vi "BenchC2_DEV.vi"() -> ()   [LabVIEW 2016]
uses:
  x64/Debug/BERTTA.dll
panel:
  out "element":bool
  out "Started:":string
  in  "SHUTDOWN":bool
  in  "MASTER CONTROL":bool
  in  "Tab Control":T1(tab)
  out "Output File":path caption="selected path"
  in  "Browse folder":path=path "" caption="start path"
  in  "Read Seq":bool
  in  "Save Seq":bool
  in  "Configuration file":path caption="Filename"
  in  "OK Button 2":bool
  out "Boolean":bool
  in  "User (initials)":string
  in  "Project name":string
  in  "Description":string
  out "PUMP1":bool
  out "Target amount":dbl
  out "Scale weight":dbl
  out "Amount now":dbl
  out "Flow rate":dbl
  out "Time to target":dbl format="%<%H:%M:%S>t"
  out "Current step":dbl
  out "Target":dbl
  out "Amount now":dbl
  out "Amount now":dbl
  out "Target":dbl
  out "Current step":dbl
  out "Time to target":dbl format="%<%H:%M:%S>t"
  out "Flow rate":dbl
  out "Amount now":dbl
  out "Scale weight":dbl
  out "Target amount":dbl
  out "PUMP2":bool
  out "Sensor OK 6":bool
  out "Sensor OK 5":bool
  out "Sensor OK 4":bool
  out "Sensor OK 3":bool
  in  "OK Button":bool
  in  "Add comment":string
  out "PUMP3":bool
  out "Target amount":dbl
  out "Scale weight":dbl
  out "Amount now":dbl
  out "Flow rate":dbl
  out "Time to target":dbl format="%<%H:%M:%S>t"
  out "Current step":dbl
  out "Target":dbl
  out "Amount now":dbl
  out "Tr":dbl
  out "Tj in":dbl
  out "Tj out":dbl
  out "T set":dbl
  out "Current step":i32
  out "RPM":dbl
  out "Torque 2":dbl
  out "Waveform Chart 5":dynamicdata(graph)
  out "Waveform Chart 6":dynamicdata(graph)
  out "Waveform Chart 7":dynamicdata(graph)
  in  "Tab Control 2":T2(tab)
  out "Waveform Chart 3":dynamicdata(graph)
  out "Waveform Chart 8":dynamicdata(graph)
  out "Waveform Chart 11":dynamicdata(graph)
  out "Waveform Chart 13":dynamicdata(graph)
  out "Waveform Chart 9":dynamicdata(graph)
  out "Table":string[][](table)=[["14.8.2017 18.06.59", "0,000000", "417,670000", "-0,150000", "1,000000", "22,220000", "23,366837", "23,574959", "23,985852", "23,690000", "240,000000", "4,000000", "0,000000", "397,000000", "-397,000000", "1,000000"], ["14.8.2017 18.07.06", "0,000000", "417,640000", "-0,120000", "1,000000", "22,220000", "23,763115", "23,906257", "23,985694", "23,680000", "240,000000", "4,000000", "0,000000", "397,000000", "-397,000000", "1,000000"], ["14.8.2017 18.07.13", "0,000000", "417,640000", "-0,120000", "1,000000", "22,220000", "23,965922", "24,013440", "23,984906", "23,670000", "240,000000", "4,100000", "3,000000", "397,000000", "-397,000000", "1,000000"], ["14.8.2017 18.07.21", "0,000000", "417,640000", "-0,120000", "1,000000", "22,220000", "23,943860", "23,900110", "23,987113", "23,670000", "240,000000", "4,000000", "0,000000", "397,000000", "-397,000000", "1,000000"], ["14.8.2017 18.07.28", "0,000000", "417,640000", "-0,120000", "1,000000", "22,220000", "23,736328", "23,600018", "23,989004", "23,660000", "240,000000", "4,000000", "0,000000", "397,000000", "-397,000000", "1,000000"], ["14.8.2017 18.07.36", "0,000000", "417,640000", "-0,120000", "1,000000", "22,220000", "23,480910", "23,324538", "23,991053", "23,660000", "240,000000", "4,000000", "0,000000", "397,000000", "-397,000000", "1,000000"], ["14.8.2017 18.07.43", "0,000000", "417,640000", "-0,120000", "2,000000", "22,220000", "23,195579", "23,008270", "23,999093", "23,650000", "240,000000", "4,000000", "0,000000", "397,000000", "-397,000000", "1,000000"], ["14.8.2017 18.07.51", "0,000000", "417,650000", "-417,650000", "1,000000", "22,220000", "22,862541", "22,649021", "24,003979", "23,650000", "240,000000", "4,000000", "0,000000", "397,000000", "-397,000000", "2,000000"], ["14.8.2017 18.07.58", "0,000000", "417,640000", "0,010000", "1,000000", "22,220000", "22,541353", "22,354878", "24,005398", "23,650000", "240,000000", "4,000000", "0,000000", "397,000000", "-397,000000", "1,000000"], ["14.8.2017 18.08.06", "0,000000", "417,640000", "0,010000", "1,000000", "22,220000", "22,347931", "22,253738", "24,007605", "23,640000", "240,000000", "4,100000", "0,000000", "397,000000", "-397,000000", "1,000000"], ["14.8.2017 18.08.13", "0,000000", "417,640000", "0,010000", "1,000000", "22,220000", "22,329030", "22,302102", "24,006028", "23,640000", "240,000000", "4,000000", "0,000000", "395,820000", "-395,820000", "1,000000"], ["14.8.2017 18.08.20", "0,000000", "417,640000", "0,010000", "1,000000", "22,220000", "22,466849", "22,511320", "24,002403", "23,630000", "240,000000", "4,000000", "0,000000", "395,830000", "-0,010000", "1,000000"], ["14.8.2017 18.08.28", "0,000000", "417,640000", "0,010000", "1,000000", "22,220000", "22,707062", "22,835101", "24,000984", "23,620000", "240,000000", "4,000000", "0,000000", "395,830000", "-0,010000", "1,000000"], ["14.8.2017 18.08.35", "0,000000", "417,640000", "0,010000", "1,000000", "22,220000", "23,054104", "23,232979", "24,001299", "23,600000", "240,000000", "4,000000", "0,000000", "395,830000", "-0,010000", "1,000000"], ["14.8.2017 18.08.43", "0,000000", "417,640000", "0,010000", "1,000000", "22,220000", "23,412371", "23,522793", "24,002560", "23,590000", "240,000000", "4,000000", "0,000000", "395,820000", "0,000000", "1,000000"], ["14.8.2017 18.08.51", "0,000000", "417,640000", "0,010000", "1,000000", "22,220000", "23,596247", "23,656125", "24,003821", "23,580000", "240,000000", "4,000000", "0,000000", "395,820000", "0,000000", "1,000000"]]
  in  "X scale":i64(slide)=50 scale=0.0..100.0
  in  "Tr/Tj mode selector 2":bool=TRUE
  in  "Tr/Tj mode selector":bool=TRUE
  out "Boolean 4":bool
  out "Boolean 3":bool
  out "Boolean 2":bool
  in  "Reset 6":bool
  in  "Manual/Ramp":bool=TRUE
  in  "Array":dbl[][](array[numeric])=[[20.0, 0.0], [20.0, 0.0], [20.0, 0.0]]
  in  "?":bool
  in  "Time":dbl format="Time to target (min):                %#_g"
  out "Current temp":dbl format="Current temperature (S1):   %#_6g"
  in  "OK Button 3":bool
  out "Sensor OK":bool
  in  "T fail":dbl=20.0 format="Failsafe temperature:              %#_g"
  in  "Setpoint":dbl=20.0 format="Temperature target:                %#_6g"
  out "Waveform Chart":dynamicdata(graph)
  out "T external 2":dbl format="Current temp S2:    %#_g"
  in  "UPDATE TEMP":bool
  out "Waveform Chart 2":dbl(graph)
  in  "Tube select":u32(ring) items=["Purple tube", "Yellow tube", " White tube"]
  out "Led11 5":bool
  out "RPM":dbl format="%_4f"
  out "Led5 3":bool
  out "Led4 3":bool
  out "Led3 3":bool
  out "Led2 3":bool
  out "Led1 3":bool
  in  "PumpSeq 4":dbl[][](array[numeric])=[[0.0, 0.0, 0.0, 0.0, 0.0, 0.0, 0.0, 0.0, 0.0, 0.0], [0.0, 0.0, 0.0, 0.0, 0.0, 0.0, 0.0, 0.0, 0.0, 0.0], [0.0, 0.0, 0.0, 0.0, 0.0, 0.0, 0.0, 0.0, 0.0, 0.0], [0.0, 0.0, 0.0, 0.0, 0.0, 0.0, 0.0, 0.0, 0.0, 0.0], [0.0, 0.0, 0.0, 0.0, 0.0, 0.0, 0.0, 0.0, 0.0, 0.0], [0.0, 0.0, 0.0, 0.0, 0.0, 0.0, 0.0, 0.0, 0.0, 0.0], [0.0, 0.0, 0.0, 0.0, 0.0, 0.0, 0.0, 0.0, 0.0, 0.0], [0.0, 0.0, 0.0, 0.0, 0.0, 0.0, 0.0, 0.0, 0.0, 0.0], [0.0, 0.0, 0.0, 0.0, 0.0, 0.0, 0.0, 0.0, 0.0, 0.0], [0.0, 0.0, 0.0, 0.0, 0.0, 0.0, 0.0, 0.0, 0.0, 0.0]]
  in  "?":bool
  out "Flow rate (g/min)":dbl
  out "Scale reading":dbl
  out "Step amount now":dbl
  in  "Grams / min":dbl
  out "Waveform Chart 14":dynamicdata(graph)
  in  "?":bool
  out "Total amount now":dbl
  out "Led11 4":bool
  in  "Reset 5":bool
  out "Elapsed / step":dbl format="%<%H:%M:%S>t"
  out "Time to target":dbl format="%<%H:%M:%S>t"
  in  "OK Button 4":bool
  out "Led11":bool
  out "RPM":dbl format="%_4f"
  out "Led10":bool
  out "Led9":bool
  out "Led8":bool
  out "Led7":bool
  out "Led6":bool
  out "Led5":bool
  out "Led4":bool
  out "Led3":bool
  out "Led2":bool
  out "Led1":bool
  in  "PumpSeq 2":dbl[][](array[numeric])=[[0.0, 0.0, 0.0, 0.0, 0.0, 0.0, 0.0, 0.0, 0.0, 0.0], [0.0, 0.0, 0.0, 0.0, 0.0, 0.0, 0.0, 0.0, 0.0, 0.0], [0.0, 0.0, 0.0, 0.0, 0.0, 0.0, 0.0, 0.0, 0.0, 0.0], [0.0, 0.0, 0.0, 0.0, 0.0, 0.0, 0.0, 0.0, 0.0, 0.0], [0.0, 0.0, 0.0, 0.0, 0.0, 0.0, 0.0, 0.0, 0.0, 0.0], [0.0, 0.0, 0.0, 0.0, 0.0, 0.0, 0.0, 0.0, 0.0, 0.0], [0.0, 0.0, 0.0, 0.0, 0.0, 0.0, 0.0, 0.0, 0.0, 0.0], [0.0, 0.0, 0.0, 0.0, 0.0, 0.0, 0.0, 0.0, 0.0, 0.0], [0.0, 0.0, 0.0, 0.0, 0.0, 0.0, 0.0, 0.0, 0.0, 0.0], [0.0, 0.0, 0.0, 0.0, 0.0, 0.0, 0.0, 0.0, 0.0, 0.0]]
  in  "?":bool
  out "Flow rate (g/min)":dbl
  out "Scale reading":dbl
  out "Step amount now":dbl
  in  "Grams / min":dbl
  out "Waveform Chart 10":dynamicdata(graph)
  in  "?":bool
  out "Total amount now":dbl
  out "Led11":bool
  in  "Reset 3":bool
  out "Elapsed / step":i32
  out "Time to target":dbl format="%<%H:%M:%S>t"
  in  "OK Button 5":bool
  out "Led11 3":bool
  out "RPM":dbl format="%_4f"
  out "Led10 2":bool
  out "Led9 2":bool
  out "Led8 2":bool
  out "Led7 2":bool
  out "Led6 2":bool
  out "Led5 2":bool
  out "Led4 2":bool
  out "Led3 2":bool
  out "Led2 2":bool
  out "Led1 2":bool
  in  "PumpSeq 3":dbl[][](array[numeric])=[[0.0, 0.0, 0.0, 0.0, 0.0, 0.0, 0.0, 0.0, 0.0, 0.0], [0.0, 0.0, 0.0, 0.0, 0.0, 0.0, 0.0, 0.0, 0.0, 0.0], [0.0, 0.0, 0.0, 0.0, 0.0, 0.0, 0.0, 0.0, 0.0, 0.0], [0.0, 0.0, 0.0, 0.0, 0.0, 0.0, 0.0, 0.0, 0.0, 0.0], [0.0, 0.0, 0.0, 0.0, 0.0, 0.0, 0.0, 0.0, 0.0, 0.0], [0.0, 0.0, 0.0, 0.0, 0.0, 0.0, 0.0, 0.0, 0.0, 0.0], [0.0, 0.0, 0.0, 0.0, 0.0, 0.0, 0.0, 0.0, 0.0, 0.0], [0.0, 0.0, 0.0, 0.0, 0.0, 0.0, 0.0, 0.0, 0.0, 0.0], [0.0, 0.0, 0.0, 0.0, 0.0, 0.0, 0.0, 0.0, 0.0, 0.0], [0.0, 0.0, 0.0, 0.0, 0.0, 0.0, 0.0, 0.0, 0.0, 0.0]]
  in  "?":bool
  out "Flow rate (g/min)":dbl
  out "Scale reading":dbl
  out "Step amount now":dbl
  in  "Grams / min":dbl
  out "Waveform Chart 12":dynamicdata(graph)
  in  "?":bool
  out "Total amount now":dbl
  out "Led11 2":bool
  in  "Reset 4":bool
  out "Elapsed / step":i32
  out "Time to target":dbl format="%<%H:%M:%S>t"
  in  "OK Button 6":bool
  in  "?":bool
  in  "Scale port":dbl=5.0
  out "Waveform Chart 15":dynamicdata(graph)
  in  "?":bool
  in  "OK Button 8":bool
  in  "Remote / Manual":bool
  in  "Set RPM":i32
  out "RPM":dbl
  out "Torque":dbl
  out "Waveform Chart 4":dynamicdata(graph)
  in  "OK Button 7":bool
  out "PortDev out":dbl[](array[numeric])
  in  "Save PortDev":bool
  out "PortDev in":dbl[](array[numeric])
  in  "dev1":i32
  in  "dev2":i32
  in  "dev3":i32
  in  "dev4":i32
  in  "dev5":i32
  in  "dev6":i32
  in  "dev8":i32
  in  "port1":i32
  in  "port2":i32
  in  "port3":i32
  in  "port4":i32
  in  "port5":i32
  in  "port6":i32
  in  "port7":i32
  in  "port8":i32
  in  "dev7":i32
  in  "Treshold (T/C)":dbl=0.5
  out "DAQ 9217 (PT100)":errorcluster
  out "Config File":dbl[][](array[numeric])
  in  "Temp Control":tag="cDAQ9188XT-1C3BF2FMod1"
  in  "PAM Control":tag="cDAQ9188XT-1C3BF2FMod7"
  # "Temperature sensor:"
  # "Manual control:"
  # "PUMP & SCALE 1"
  # "STEP"
  # "TOTAL"
  # "PUMP & SCALE 2"
  # "STEP"
  # "TOTAL"
  # "PUMP & SCALE 3"
  # "STEP"
  # "TOTAL"
  # "Temperature control parameter"
  # "Secondary temperature sensor"
  # "Temp target"
  # "Time target"
  # "Grams    /   min"
  # "End of sequence"
  # "Manual control"
  # "Grams    /   min"
  # "End of sequence"
  # "Manual control"
  # "Grams    /   min"
  # "End of sequence"
  # "Manual control"
  # "PAM control"
  # "dev1 and dev2 always to port1 and 2\nport1 = port2 = Lauda\n\ndev3 and dev4 always to port3 and port4\nport3 = port4 = Heidolph"
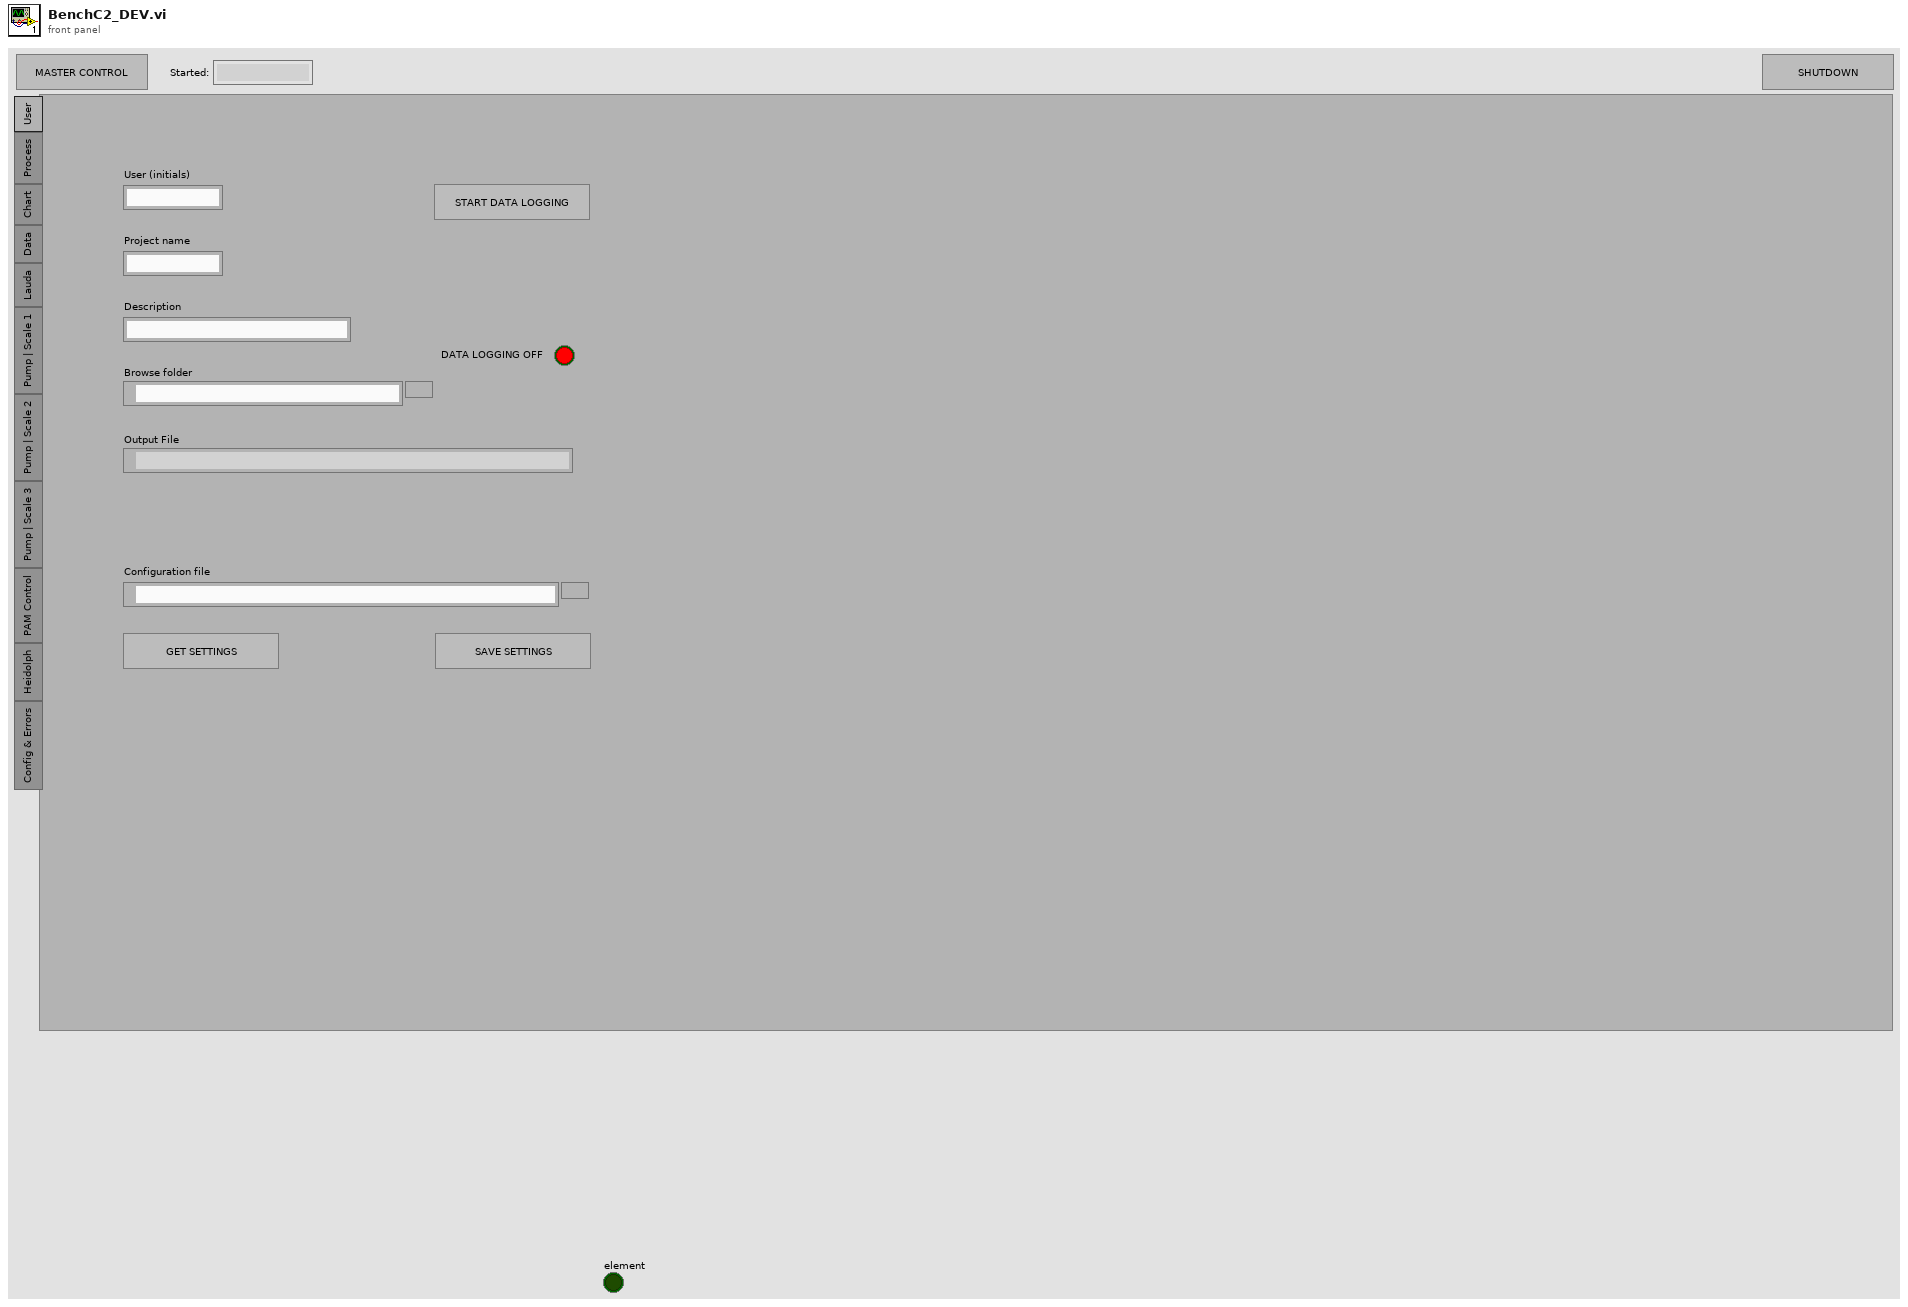
[diagram p1: front panel]
types:
  T1 = enum32{"User", "Process", "Chart", "Data", "Lauda", "Pump | Scale 1", "Pump | Scale 2", "Pump | Scale 3", "PAM Control", "Heidolph", "Config & Errors"}
  T2 = enum32{"Temperatures", "Scale / Pump 1", "Scale / Pump 2", "Scale / Pump 3", "RPM / torque"}
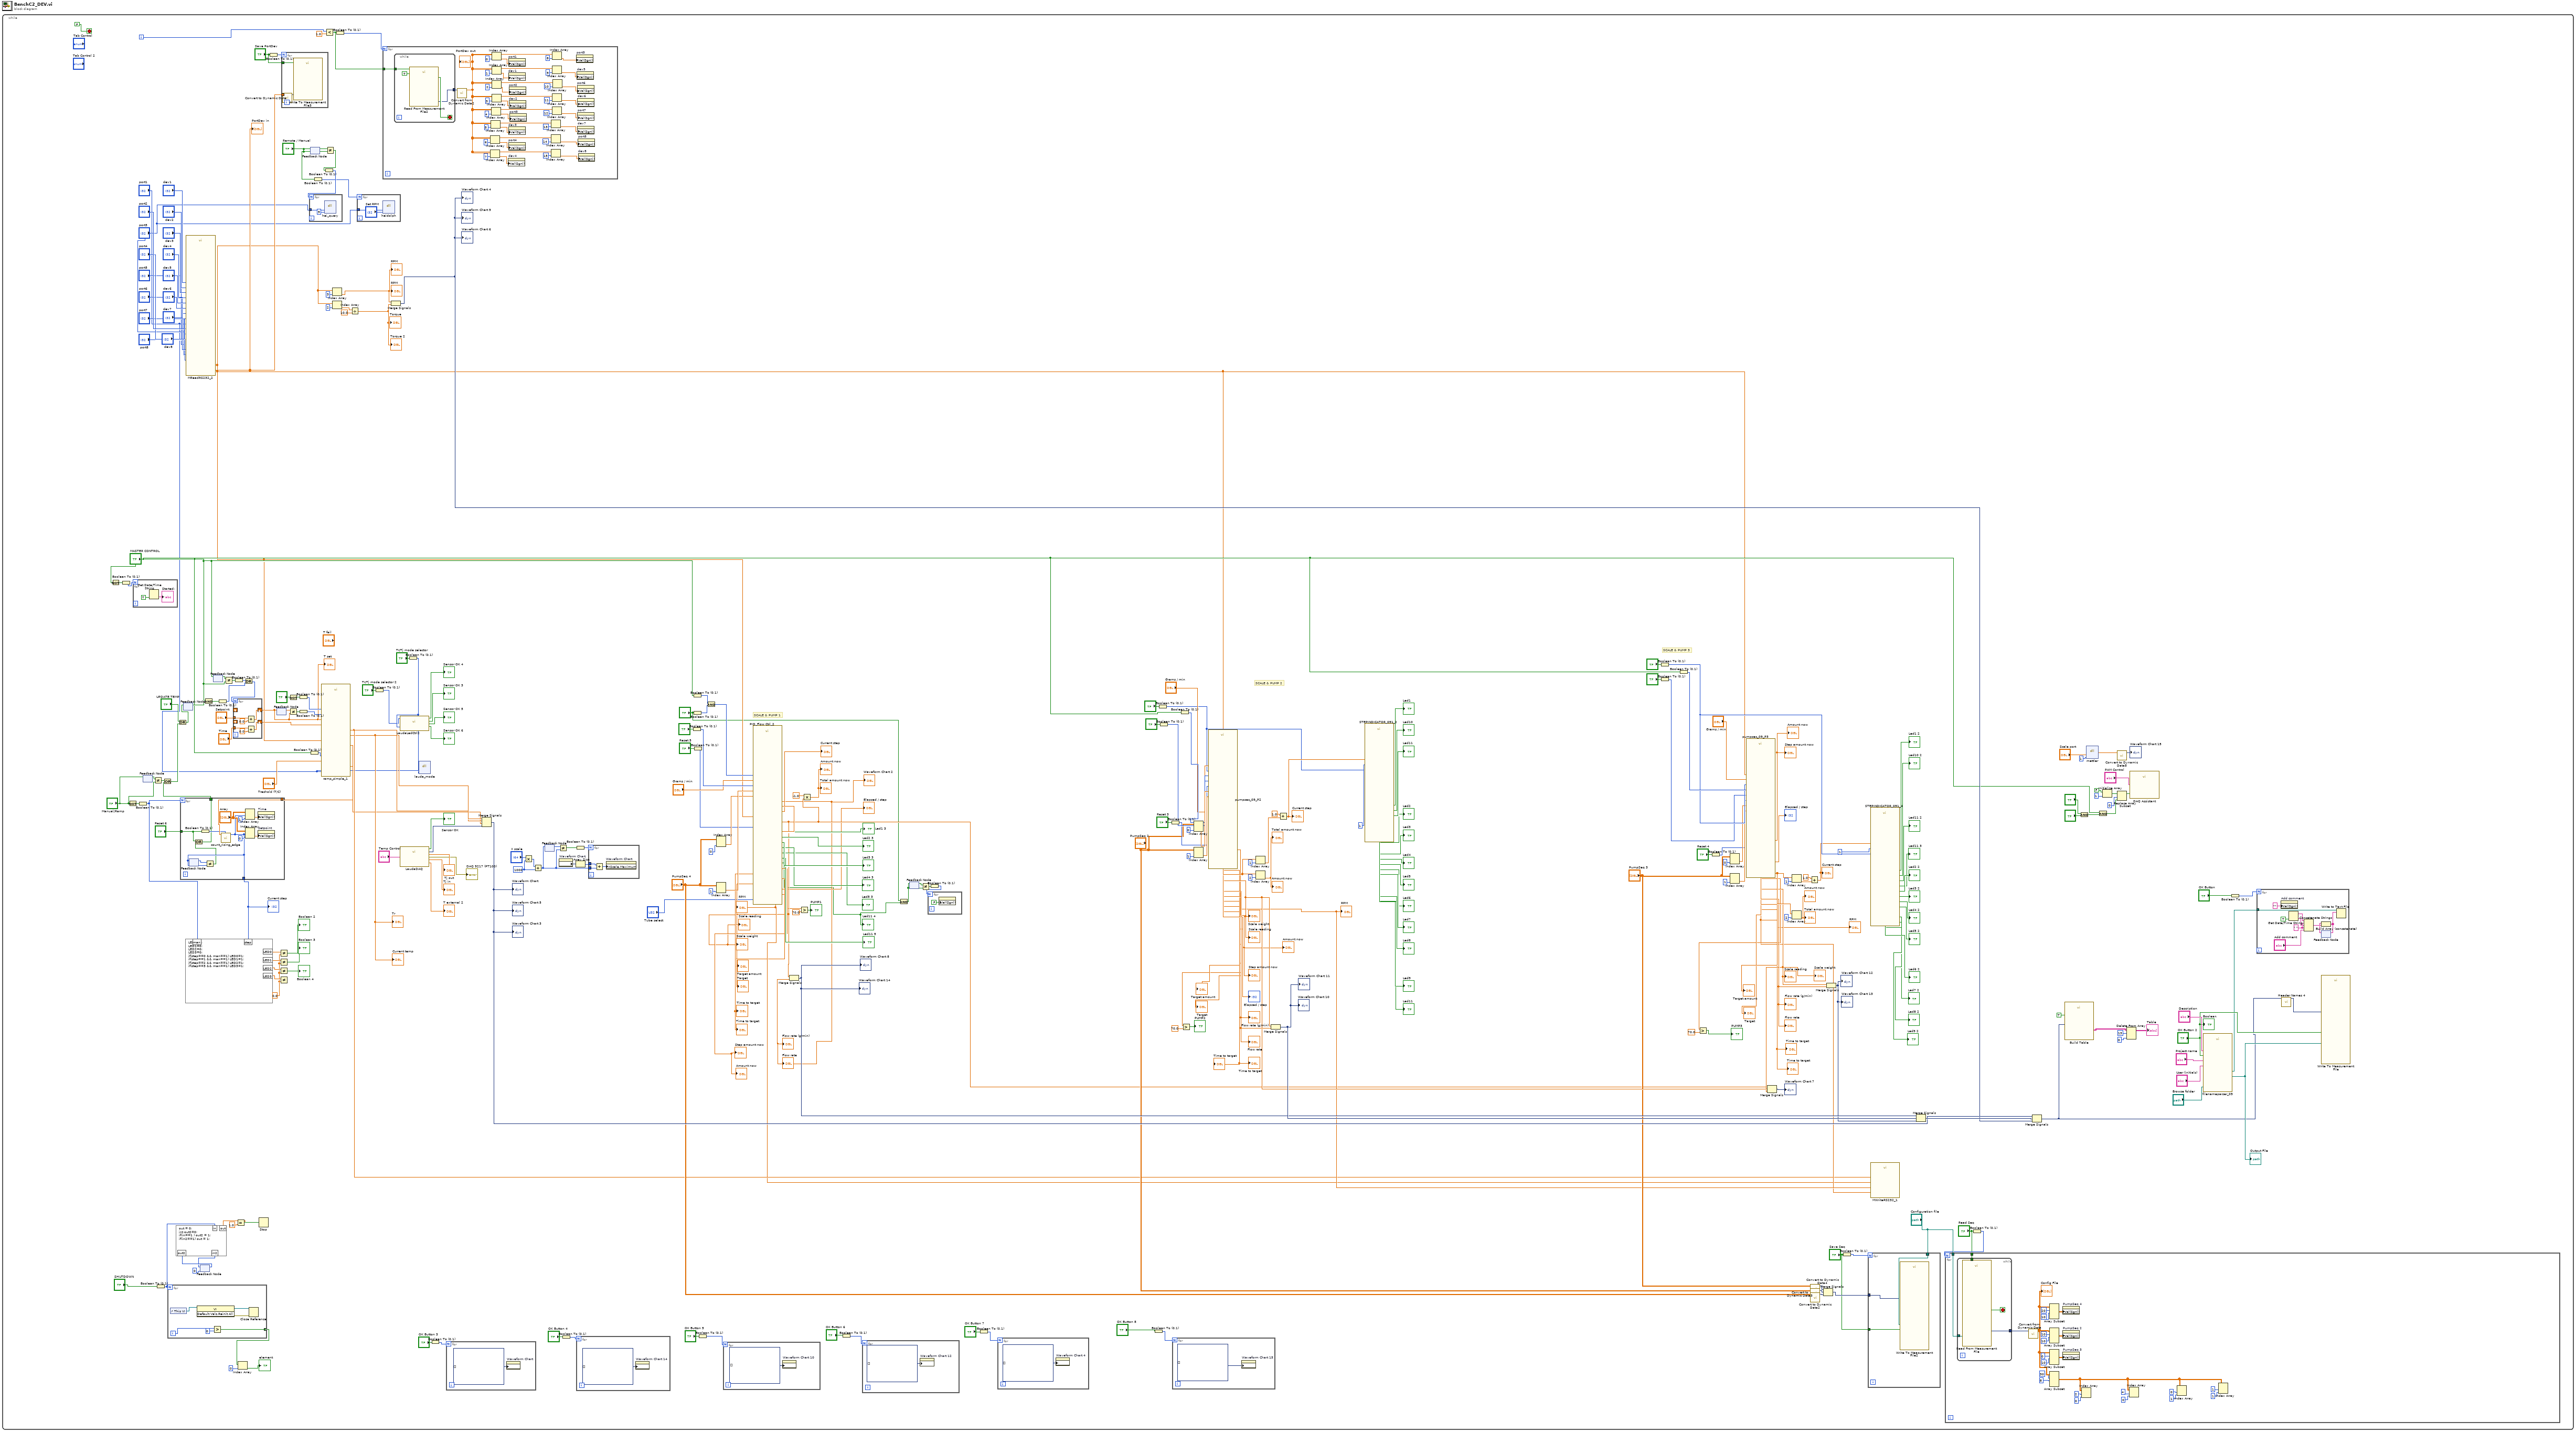
[diagram p0: block diagram]
diagram:
  n1 = while {
    i -> [w110]
    stop <- FALSE stop-if-true
    w42 = i64 1000 ("y")
    w96 = 0.0 ("y")
    # "SCALE & PUMP 1"
    # "SCALE & PUMP 3"
    # "SCALE & PUMP 2"
    n2 = Not(x="MASTER CONTROL") -> (.not. x?=w297:bool)
    n3 = Boolean To (0,1)(Boolean=w297) -> (0, 1=w298:i16)
    n4 = Not(x="Manual/Ramp") -> (.not. x?=w103:bool)
    n5 = for {
      N: w298 -> [_]
      n6 = Get Date/Time String(want seconds? (F)=TRUE) -> (time string=→"Started:":string)  [unwired: 2 in, 1 out]
    }
    n7 = Boolean To (0,1)(Boolean=w103) -> (0, 1=w86:i16)
    n8 = feedback #1() -> (w92:bool)  [unwired: 1 in]
    n9 = feedback-in #1("Manual/Ramp") -> ()
    n10 = Not Equal?(x=w92, y="Manual/Ramp") -> (x != y?=w89:bool)
    n11 = Boolean To (0,1)(Boolean="SHUTDOWN") -> (0, 1=w282:i16)
    n12 = for {
      N: w282 -> [_]
      tunnel: [w418] -> w296 mode=indexing
      i -> [w420]
      n13 = control-ref of="This VI"() -> (w423:refnum<vi>)
      n14 = invoke class="VI" method="Default Vals.Reinit All"(reference=w423) -> (reference out=w421:refnum<vi>, error out=w422:errorcluster)  [unwired: 2 in, 1 out]
      n15 = Greater?(x=w420, y=0) -> (0:w418:bool)
      n16 = Close Reference(reference=w421, error in (no error)=w422) -> ()  [unwired: 1 out]
    }
    n17 = feedback #2() -> (w84:bool)  [unwired: 1 in]
    n18 = call "MReadRS232_2.vi"("port1"="port1", "dev1"="dev1", "port2"="port2", "dev2"="dev2", "port3"="port3", "dev7"="dev7", "dev8"="dev8", "port7"="port7", "port8"="port8", "dev5"="dev5", "port5"="port5", "dev4"="dev4", "dev6"="dev6", "port6"="port6", "port4"="port4", "dev3"="dev3") -> ("output array"=w114:dbl[], "params"=w30:dbl[])  [unwired: 2 in]
    "PortDev in" <- w114
    n19 = feedback #3(0) -> (w280:i32)
    n20 = formula code="out = 0;\nint out2=0;\nif(in==1 ) out2 = 1;\nif(in2==1) out = 1;"("in"=w282, "in2"=w280) -> ("out"=w284:dbl, "out2"=w281:i32)
    n21 = feedback-in #3(w281) -> ()
    n22 = And(x="MASTER CONTROL", y=w84) -> (x .and. y?=w140:bool)
    n23 = feedback #4() -> (w132:bool)  [unwired: 1 in]
    n24 = feedback-in #4("MASTER CONTROL") -> ()
    n25 = Boolean To (0,1)(Boolean=w140) -> (0, 1=w130:i16)
    n26 = Not Equal?(x=w132, y="MASTER CONTROL") -> (x != y?=w131:bool)
    n27 = Boolean To (0,1)(Boolean=w131) -> (0, 1=w129:i16)
    n28 = Equal?(x=w284, y=1.0) -> (x = y?=w283:bool)
    n29 = Index Array(array=w296, index=0) -> (element=→"element":bool)
    n30 = Or(x=w129, y=w130) -> (x .or. y?=w128:i16)
    n31 = for {
      N: w128 -> [_]
      tunnel: "Time" -> [w370]
      shift-right: [w369] -> w141
      shift-left: _ -> [_]
      tunnel: "Setpoint" -> [w367]
      shift-right: [w366] -> w51
      shift-left: _ -> [_]
      n32 = Add(x=w367, y=0.0) -> (x+y=w366:dbl)
      n33 = Add(x=w370, y=0.0) -> (x+y=w369:dbl)
    }
    "T set" <- w51
    n34 = Stop(stop? (T)=w283) -> ()
    n35 = Boolean To (0,1)(Boolean="Save PortDev") -> (0, 1=w113:i16)
    n36 = feedback-in #5(w51) -> ()
    n37 = feedback #5() -> (w139:dbl)  [unwired: 1 in]
    n38 = for {
      N: w113 -> [_]
      tunnel: w114 -> [w365]
      tunnel: "Save PortDev" -> [w363]
      n39 = call "Convert to Dynamic Data"("Array"=w365) -> ("Dynamic Data Type"=w364:dynamicdata)  [unwired: 3 in]
      n40 = call "Write To Measurement File3"("Signals"=w364, "Reset"=w363) -> ()  [unwired: 15 in, 3 out]
    }
    n41 = Not(x="?") -> (.not. x?=w135:bool)
    n42 = Not Equal?(x=w139, y=w51) -> (x != y?=w138:bool)
    n43 = Boolean To (0,1)(Boolean=w135) -> (0, 1=w137:i16)
    n44 = Boolean To (0,1)(Boolean=w138) -> (0, 1=w133:i16)
    n45 = Boolean To (0,1)(Boolean="MASTER CONTROL") -> (0, 1=w134:i16)
    n46 = feedback-in #6("Remote / Manual") -> ()
    n47 = feedback #6() -> (w81:bool)  [unwired: 1 in]
    n48 = Boolean To (0,1)(Boolean="Remote / Manual") -> (0, 1=w79:i16)
    n49 = call "ramp_simple_1.vi"("pause"=w137, "time_set"=w141, "array"=w30, "reset"=w133, "master"=w134, "T_sp"=w51, "treshold"="Treshold (T/C)", "port"="port1") -> ("Tin"=w144:dbl, "Tr"=w145:dbl, "target_reached"=w101:dbl, "T control"=w146:dbl)  [unwired: 3 in, 1 out]
    "Tr" <- w145
    "Current temp" <- w145
    n50 = for {
      N: w86 -> [_]
      tunnel: w101 -> [w322]
      tunnel: [w312] -> w90
      tunnel: "Reset 6" -> [w314]
      tunnel: [w315] -> w52
      n51 = feedback #7() -> (w316:i32)  [unwired: 1 in]
      n52 = Boolean To (0,1)(Boolean=w314) -> (0, 1=w317:i16)
      n53 = call "count_rising_edge.vi"("reset"=w317, "target_reached"=w322) -> ("element 2"=w315:i32)  [unwired: 9 in]
      n54 = feedback-in #7(w315) -> ()
      n55 = Not Equal?(x=w316, y=w315) -> (x != y?=w313:bool)
      n56 = Or(x=w314, y=w313) -> (x .or. y?=w312:bool)
      n57 = Index Array(array="Array", index (row)=w315, index (col)=1 ("disabled index (col)")) -> (element=w318:dbl)
      n58 = Index Array(array="Array", index (row)=w315, index (col)=0 ("disabled index (col)")) -> (element=w319:dbl)
      n59 = property on="Time" class="DigNum (strict)"("Val(Sgnl)"=w318) -> ()  [unwired: 2 in, 2 out]
      n60 = property on="Setpoint" class="DigNum (strict)"("Val(Sgnl)"=w319) -> ()  [unwired: 2 in, 2 out]
    }
    "Current step" <- w52
    n61 = Or(x=w89, y=w90) -> (x .or. y?=w88:bool)
    n62 = Or(x="UPDATE TEMP", y=w88) -> (x .or. y?=w85:bool)
    n63 = feedback-in #2(w85) -> ()
    n64 = formula code="LED0=0;\nLED1=0;\nLED2=0;\nLED3=0;\nif(step==0 && man==1) LED0=1;\nif(step==1 && man==1) LED1=1;\nif(step==2 && man==1) LED2=1;\nif(step==3 && man==1) LED3=1;"("step"=w52, "man"=w86) -> ("LED0"=w100:dbl, "LED1"=w99:dbl, "LED2"=w98:dbl, "LED3"=w97:dbl)
    n65 = Not Equal?(x=w100, y=w96) -> (x != y?=→"Boolean 2":bool)
    n66 = Not Equal?(x=w99, y=w96) -> (x != y?=→"Boolean 3":bool)
    n67 = Not Equal?(x=w98, y=w96) -> (x != y?=→"Boolean 4":bool)
    n68 = Not Equal?(x=w97, y=w96) -> ()  [unwired: 1 out]
    n69 = Less?(x=w110, y=1.0) -> (x < y?=w108:bool)
    n70 = Not Equal?(x=w81, y="Remote / Manual") -> (x != y?=w80:bool)
    n71 = Boolean To (0,1)(Boolean=w80) -> (0, 1=w82:i16)
    n72 = for {
      N: w82 -> [_]
      tunnel: "port3" -> [w310]
      n73 = dll-call lib="C:/Users/shresplab/OneDrive - Kemira Oyj/Documents/GitHub/Bertta/BERTTA/x64/Debug/BERTTA.dll" fn="hei_query"("port"=w310, "q"=5) -> ()  [unwired: 6 in, 2 out]
    }
    n74 = Index Array(array=w30, index=3) -> (element=w74:dbl)
    "RPM" <- w74
    "RPM" <- w74
    n75 = Index Array(array=w30, index=2) -> (element=w76:dbl)
    n76 = Boolean To (0,1)(Boolean=w108) -> (0, 1=w109:i16)
    n77 = Divide(x=w76, y=10.0) -> (x/y=w73:dbl)
    "Torque" <- w73
    "Torque 2" <- w73
    n78 = for {
      N: w79 -> [_]
      tunnel: "port3" -> [w308]
      n79 = dll-call lib="C:/Users/shresplab/OneDrive - Kemira Oyj/Documents/GitHub/Bertta/BERTTA/x64/Debug/BERTTA.dll" fn="heidolph"("port"=w308, "speed"="Set RPM") -> ()  [unwired: 6 in, 2 out]
    }
    n80 = Boolean To (0,1)(Boolean="Tr/Tj mode selector 2") -> (0, 1=w46:i16)
    n81 = for {
      N: w109 -> [_]
      tunnel: w108 -> [w358]
      n82 = while {
        tunnel: [w361] -> w357
        tunnel: w358 -> [w359]
        stop <- w362 stop-if-true
        n83 = call "Read From Measurement File2"("Enable"=TRUE, "Reset"=w359) -> ("Signals"=w361:dynamicdata, "EOF?"=w362:bool)  [unwired: 4 in, 4 out]
      }
      n84 = call "Convert from Dynamic Data2"("Dynamic Data Type"=w357) -> ("Array"=w340:dbl[])  [unwired: 3 in]
      "PortDev out" <- w340
      n85 = Index Array(array=w340, index=6) -> (element=w333:dbl)
      n86 = Index Array(array=w340, index=7) -> (element=w332:dbl)
      n87 = Index Array(array=w340, index=5) -> (element=w334:dbl)
      n88 = Index Array(array=w340, index=4) -> (element=w335:dbl)
      n89 = Index Array(array=w340, index=0) -> (element=w339:dbl)
      n90 = Index Array(array=w340, index=1) -> (element=w338:dbl)
      n91 = Index Array(array=w340, index=3) -> (element=w336:dbl)
      n92 = Index Array(array=w340, index=2) -> (element=w337:dbl)
      n93 = property on="dev4" class="DigNum (strict)"("Val(Sgnl)"=w332) -> ()  [unwired: 2 in, 2 out]
      n94 = property on="dev3" class="DigNum (strict)"("Val(Sgnl)"=w334) -> ()  [unwired: 2 in, 2 out]
      n95 = property on="port4" class="DigNum (strict)"("Val(Sgnl)"=w333) -> ()  [unwired: 2 in, 2 out]
      n96 = property on="port1" class="DigNum (strict)"("Val(Sgnl)"=w339) -> ()  [unwired: 2 in, 2 out]
      n97 = property on="dev1" class="DigNum (strict)"("Val(Sgnl)"=w338) -> ()  [unwired: 2 in, 2 out]
      n98 = property on="port2" class="DigNum (strict)"("Val(Sgnl)"=w337) -> ()  [unwired: 2 in, 2 out]
      n99 = property on="dev2" class="DigNum (strict)"("Val(Sgnl)"=w336) -> ()  [unwired: 2 in, 2 out]
      n100 = property on="port3" class="DigNum (strict)"("Val(Sgnl)"=w335) -> ()  [unwired: 2 in, 2 out]
      n101 = Index Array(array=w340, index=14) -> (element=w325:dbl)
      n102 = Index Array(array=w340, index=15) -> (element=w324:dbl)
      n103 = Index Array(array=w340, index=13) -> (element=w326:dbl)
      n104 = Index Array(array=w340, index=12) -> (element=w327:dbl)
      n105 = Index Array(array=w340, index=8) -> (element=w331:dbl)
      n106 = Index Array(array=w340, index=9) -> (element=w330:dbl)
      n107 = Index Array(array=w340, index=11) -> (element=w328:dbl)
      n108 = Index Array(array=w340, index=10) -> (element=w329:dbl)
      n109 = property on="port5" class="DigNum (strict)"("Val(Sgnl)"=w331) -> ()  [unwired: 2 in, 2 out]
      n110 = property on="dev5" class="DigNum (strict)"("Val(Sgnl)"=w330) -> ()  [unwired: 2 in, 2 out]
      n111 = property on="port6" class="DigNum (strict)"("Val(Sgnl)"=w329) -> ()  [unwired: 2 in, 2 out]
      n112 = property on="dev6" class="DigNum (strict)"("Val(Sgnl)"=w328) -> ()  [unwired: 2 in, 2 out]
      n113 = property on="port7" class="DigNum (strict)"("Val(Sgnl)"=w327) -> ()  [unwired: 2 in, 2 out]
      n114 = property on="dev7" class="DigNum (strict)"("Val(Sgnl)"=w326) -> ()  [unwired: 2 in, 2 out]
      n115 = property on="port8" class="DigNum (strict)"("Val(Sgnl)"=w325) -> ()  [unwired: 2 in, 2 out]
      n116 = property on="dev8" class="DigNum (strict)"("Val(Sgnl)"=w324) -> ()  [unwired: 2 in, 2 out]
    }
    n117 = Merge Signals(w74, w73) -> (w72:dynamicdata)
    "Waveform Chart 4" <- w72
    "Waveform Chart 6" <- w72
    "Waveform Chart 9" <- w72
    n118 = call "LaudaDAQ.vi"("device name"="Temp Control") -> ("error out"=→"DAQ 9217 (PT100)":errorcluster, 1:"Tj out"=→"Tj out":dbl, "data"=w202:dynamicdata, "Sensor OK"=→"Sensor OK":bool, 4:"Tj out"=→"Tj in":dbl, "T external 2"=→"T external 2":dbl)  [unwired: 5 in]
    n119 = Boolean To (0,1)(Boolean="Tr/Tj mode selector") -> (0, 1=w48:i16)
    n120 = call "LaudaLedCtrl2.vi"("ctrl_mode"=w48, "T ext / T ext in"=w46) -> ("Sensor OK 5"=→"Sensor OK 5":bool, "Sensor OK 3"=→"Sensor OK 3":bool, "Sensor OK 4"=→"Sensor OK 4":bool, "Sensor OK 6"=→"Sensor OK 6":bool)  [unwired: 6 in]
    n121 = dll-call lib="C:/Users/shresplab/OneDrive - Kemira Oyj/Documents/GitHub/Bertta/BERTTA/x64/Debug/BERTTA.dll" fn="lauda_mode"("port"="port1", "mode"=w48) -> ()  [unwired: 6 in, 2 out]
    n122 = Boolean To (0,1)(Boolean="OK Button 3") -> (0, 1=w157:i16)
    n123 = for {
      N: w157 -> [_]
      n124 = property on="Waveform Chart" class="WFChart (strict)"("History Data"=dynamicdata[] []) -> ()  [unwired: 2 in, 2 out]
    }
    n125 = Merge Signals(w146, w145, w144, w202) -> (w203:dynamicdata)
    "Waveform Chart 3" <- w203
    "Waveform Chart" <- w203
    "Waveform Chart 5" <- w203
    n126 = Multiply(x="X scale", y=w42) -> (x*y=w43:i64)
    n127 = Add(x=w43, y=w42) -> (x+y=w38:i64)
    n128 = feedback-in #8(w38) -> ()
    n129 = feedback #8() -> (w41:i64)  [unwired: 1 in]
    n130 = Not Equal?(x=w41, y=w38) -> (x != y?=w40:bool)
    n131 = property on="Waveform Chart" class="WFChart (strict)"() -> ("History Data"=w45:dynamicdata[])  [unwired: 2 in, 2 out]
    n132 = Boolean To (0,1)(Boolean="OK Button 4") -> (0, 1=w155:i16)
    n133 = Boolean To (0,1)(Boolean=w40) -> (0, 1=w37:i16)
    n134 = Array Size(array=w45) -> (size(s)=w39:i32)
    n135 = for {
      N: w155 -> [_]
      n136 = property on="Waveform Chart 14" class="WFChart (strict)"("History Data"=dynamicdata[] []) -> ()  [unwired: 2 in, 2 out]
    }
    n137 = for {
      N: w37 -> [_]
      tunnel: w39 -> [w306]
      tunnel: w38 -> [w305]
      n138 = Add(x=w306, y=w305) -> (x+y=w304:i64)
      n139 = property on="Waveform Chart" class="WFChart (strict)"("XScale.Maximum"=w304) -> ()  [unwired: 2 in, 2 out]
    }
    n140 = Boolean To (0,1)(Boolean="?") -> (0, 1=w36:i16)
    n141 = Boolean To (0,1)(Boolean="?") -> (0, 1=w7:i16)
    n142 = Boolean To (0,1)(Boolean="MASTER CONTROL") -> (0, 1=w34:i16)
    n143 = Boolean To (0,1)(Boolean="Reset 5") -> (0, 1=w28:i16)
    n144 = Boolean To (0,1)(Boolean="OK Button 5") -> (0, 1=w153:i16)
    n145 = And(x=w34, y=w7) -> (x .and. y?=w33:i16)
    n146 = Index Array(array="PumpSeq 4", index (col)=0) -> (element=w31:dbl[])  [unwired: 1 in]
    n147 = Index Array(array="PumpSeq 4", index (col)=1) -> (element=w32:dbl[])  [unwired: 1 in]
    n148 = for {
      N: w153 -> [_]
      n149 = property on="Waveform Chart 10" class="WFChart (strict)"("History Data"=dynamicdata[] []) -> ()  [unwired: 2 in, 2 out]
    }
    n150 = call "PID_Flow Ctrl_2.vi"("weight"=w30, "Setpoint_W"=w31, "Setpoint_T"=w32, "FrManual"="Grams / min", "enable"=w33, "manual"=w36, "reset"=w28, "tube"="Tube select") -> ("elapsed_step"=→"Elapsed / step":dbl, "total_target"=→"Target":dbl, "Setpoint_W"=→"Target amount":dbl, "LED_stop"=w6:bool, "RPM"=w29:dbl, "LED1"=→"Led1 3":bool, "LED4"=→"Led4 3":bool, "LED2"=→"Led2 3":bool, "step_amount"=→"Amount now" →"Step amount now":dbl, "LED3"=→"Led3 3":bool, "LED5"=→"Led5 3":bool, "weight"=w17:dbl, "time_to_target"=→"Time to target" →"Time to target":dbl, "PumpCTRL"=w11:dbl, "step"=→"Current step":dbl, "LED_manual"=→"Led11 5":bool, "FR"=w8:dbl)  [unwired: 3 in]
    "Flow rate" <- w8
    "Scale weight" <- w17
    "Led11 4" <- w6
    "Scale reading" <- w17
    "Flow rate (g/min)" <- w8
    "RPM" <- w29
    "Waveform Chart 2" <- w8
    n151 = Merge Signals(w17, w8) -> (w206:dynamicdata)
    "Waveform Chart 8" <- w206
    "Waveform Chart 14" <- w206
    n152 = Greater?(x=w11, y=70.0) -> (0:→"PUMP1":bool)
    n153 = Multiply(x=-1.0, y=w17) -> (x*y=→"Amount now" →"Total amount now":dbl)
    n154 = Boolean To (0,1)(Boolean="OK Button 6") -> (0, 1=w151:i16)
    n155 = for {
      N: w151 -> [_]
      n156 = property on="Waveform Chart 12" class="WFChart (strict)"("History Data"=dynamicdata[] []) -> ()  [unwired: 2 in, 2 out]
    }
    n157 = And(x="?", y=w6) -> (x .and. y?=w3:bool)
    n158 = feedback #9() -> (w4:bool)  [unwired: 1 in]
    n159 = feedback-in #9(w3) -> ()
    n160 = Not Equal?(x=w4, y=w3) -> (x != y?=w2:bool)
    n161 = Boolean To (0,1)(Boolean=w2) -> (0, 1=w1:i16)
    n162 = for {
      N: w1 -> [_]
      n163 = property class="Bool (strict)"("Val(Sgnl)"=FALSE ("Value (Signaling)")) -> ()  [unwired: 2 in, 2 out]
    }
    n164 = Boolean To (0,1)(Boolean="OK Button 7") -> (0, 1=w149:i16)
    n165 = for {
      N: w149 -> [_]
      n166 = property on="Waveform Chart 4" class="WFChart (strict)"("History Data"=dynamicdata[] []) -> ()  [unwired: 2 in, 2 out]
    }
    n167 = Boolean To (0,1)(Boolean="OK Button 8") -> (0, 1=w69:i16)
    n168 = Boolean To (0,1)(Boolean="?") -> (0, 1=w246:i16)
    n169 = Boolean To (0,1)(Boolean="?") -> (0, 1=w272:i16)
    n170 = Boolean To (0,1)(Boolean="Reset 3") -> (0, 1=w270:i16)
    n171 = for {
      N: w69 -> [_]
      n172 = property on="Waveform Chart 15" class="WFChart (strict)"("History Data"=dynamicdata[] []) -> ()  [unwired: 2 in, 2 out]
    }
    n173 = Boolean To (0,1)(Boolean="MASTER CONTROL") -> (0, 1=w264:i16)
    n174 = Index Array(array="PumpSeq 2", index (col)=0 ("disabled index (col)")) -> (element=w275:dbl[])  [unwired: 1 in]
    n175 = Index Array(array="PumpSeq 2", index (col)=1 ("disabled index (col)")) -> (element=w274:dbl[])  [unwired: 1 in]
    n176 = call "pumpsec_09_P2.vi"("reset"=w270, "master"=w264, "manual"=w246, "pause"=w272, "Array"=w30, "Target"=w275, "fr_manual"="Grams / min", "Time"=w274) -> ("pumpCtrl"=w189:dbl, "totaltarget"=→"Target":dbl, "target_step"=→"Target amount":dbl, "REGLO D"=w162:dbl, "time_to_target"=→"Time to target" →"Time to target":dbl, "step_fr"=w201:dbl, "amount_step"=→"Amount now" →"Step amount now":dbl, "Scale"=w198:dbl, "elapsed_step"=→"Elapsed / step":dbl, "params"=w265:dbl[])  [unwired: 8 in, 2 out]
    "Scale weight" <- w198
    "Flow rate" <- w201
    "Scale reading" <- w198
    "Flow rate (g/min)" <- w201
    "RPM" <- w162
    n177 = Greater?(x=w189, y=70.0) -> (0:→"PUMP2":bool)
    n178 = Index Array(array=w265, index=1) -> (element=w268:dbl)
    n179 = Index Array(array=w265, index=2) -> (element=→"Amount now" →"Total amount now":dbl)
    n180 = Merge Signals(w198, w201) -> (w207:dynamicdata)
    "Waveform Chart 11" <- w207
    "Waveform Chart 10" <- w207
    n181 = Add(x=1.0, y=w268) -> (x+y=w262:dbl)
    "Current step" <- w262
    n182 = call "STEPINDICATOR_091_2.vi"("current step"=w262, "enable"=i16 1, "manual"=w246) -> ("Led 8"=→"Led8":bool, "Led 10"=→"Led10":bool, "Led 11"=→"Led11":bool, "Led 7"=→"Led7":bool, "Led 1"=→"Led1":bool, "Led 6"=→"Led6":bool, "Led 2"=→"Led2":bool, "Led 12"=→"Led11":bool, "Led 5"=→"Led5":bool, "Led 4"=→"Led4":bool, "Led 3"=→"Led3":bool, "Led 9"=→"Led9":bool)  [unwired: 1 in]
    n183 = Boolean To (0,1)(Boolean="?") -> (0, 1=w240:i16)
    n184 = Boolean To (0,1)(Boolean="?") -> (0, 1=w239:i16)
    n185 = Boolean To (0,1)(Boolean="MASTER CONTROL") -> (0, 1=w241:i16)
    n186 = Boolean To (0,1)(Boolean="Reset 4") -> (0, 1=w221:i16)
    n187 = Index Array(array="PumpSeq 3", index (col)=0 ("disabled index (col)")) -> (element=w224:dbl[])  [unwired: 1 in]
    n188 = Index Array(array="PumpSeq 3", index (col)=1 ("disabled index (col)")) -> (element=w223:dbl[])  [unwired: 1 in]
    n189 = call "pumpsec_09_P3.vi"("reset"=w221, "master"=w241, "manual"=w240, "pause"=w239, "Array"=w30, "Target"=w224, "fr_manual"="Grams / min", "Time"=w223) -> ("pumpCtrl"=w186:dbl, "totaltarget"=→"Target":dbl, "target_step"=→"Target amount":dbl, "REGLO D"=w161:dbl, "time_to_target"=→"Time to target" →"Time to target":dbl, "step_fr"=w200:dbl, "amount_step"=→"Amount now" →"Step amount now":dbl, "Scale"=w197:dbl, "elapsed_step"=→"Elapsed / step":dbl, "params"=w214:dbl[])  [unwired: 8 in, 2 out]
    "Scale weight" <- w197
    "Flow rate" <- w200
    "Scale reading" <- w197
    "Flow rate (g/min)" <- w200
    "RPM" <- w161
    n190 = Greater?(x=w186, y=70.0) -> (0:→"PUMP3":bool)
    n191 = Merge Signals(w17, w198, w197) -> (→"Waveform Chart 7":dynamicdata)
    n192 = Index Array(array=w214, index=1) -> (element=w215:dbl)
    n193 = Index Array(array=w214, index=2) -> (element=→"Amount now" →"Total amount now":dbl)
    n194 = Add(x=1.0, y=w215) -> (x+y=w213:dbl)
    "Current step" <- w213
    n195 = call "Convert to Dynamic Data4"("2D Array"="PumpSeq 3") -> ("Dynamic Data Type"=w165:dynamicdata)  [unwired: 3 in]
    n196 = call "Convert to Dynamic Data3"("2D Array"="PumpSeq 2") -> ("Dynamic Data Type"=w167:dynamicdata)  [unwired: 3 in]
    n197 = call "Convert to Dynamic Data2"("2D Array"="PumpSeq 4") -> ("Dynamic Data Type"=w170:dynamicdata)  [unwired: 3 in]
    n198 = Merge Signals(w165, w167, w170) -> (w169:dynamicdata)
    n199 = Merge Signals(w197, w200) -> (w205:dynamicdata)
    "Waveform Chart 13" <- w205
    "Waveform Chart 12" <- w205
    n200 = Boolean To (0,1)(Boolean="Save Seq") -> (0, 1=w164:i16)
    n201 = for {
      N: w164 -> [_]
      tunnel: w169 -> [w416]
      tunnel: "Configuration file" -> [w417]
      tunnel: "Save Seq" -> [w415]
      n202 = call "Write To Measurement File2"("Signals"=w416, "Reset"=w415, "Filename"=w417) -> ()  [unwired: 14 in, 3 out]
    }
    n203 = call "STEPINDICATOR_091_4.vi"("current step"=w213, "enable"=i16 1, "manual"=w240) -> ("Led 8"=→"Led8 2":bool, "Led 10"=→"Led10 2":bool, "Led 11"=→"Led11 2":bool, "Led 7"=→"Led7 2":bool, "Led 1"=→"Led1 2":bool, "Led 6"=→"Led6 2":bool, "Led 2"=→"Led2 2":bool, "Led 12"=→"Led11 3":bool, "Led 5"=→"Led5 2":bool, "Led 4"=→"Led4 2":bool, "Led 3"=→"Led3 2":bool, "Led 9"=→"Led9 2":bool)  [unwired: 1 in]
    n204 = call "MWriteRS232_1.vi"("P3"=w161, "P2"=w162, "P1"=w29, "LAUDA"=w146) -> ()  [unwired: 8 in]
    n205 = Merge Signals(w206, w207, w205) -> (w204:dynamicdata)
    n206 = Boolean To (0,1)(Boolean="Read Seq") -> (0, 1=w163:i16)
    n207 = for {
      N: w163 -> [_]
      tunnel: "Configuration file" -> [w388]
      tunnel: "Read Seq" -> [w387]
      n208 = while {
        tunnel: [w414] -> w410
        tunnel: w388 -> [w413]
        tunnel: w387 -> [w411]
        stop <- w412 stop-if-true
        n209 = call "Read From Measurement File"("Filename"=w413, "Reset"=w411) -> ("Signals"=w414:dynamicdata, "EOF?"=w412:bool)  [unwired: 4 in, 4 out]
      }
      n210 = call "Convert from Dynamic Data"("Dynamic Data Type"=w410) -> ("Array"=w400:dbl[][])  [unwired: 3 in]
      "Config File" <- w400
      n211 = Array Subset(array=w400, index (row)=20 ("index"), length (row)=10 ("length")) -> (w407:dbl[][])  [unwired: 2 in]
      n212 = Array Subset(array=w400, index (row)=10 ("index"), length (row)=10 ("length")) -> (w402:dbl[][])  [unwired: 2 in]
      n213 = Array Subset(array=w400, index (row)=0 ("index"), length (row)=10 ("length")) -> (w401:dbl[][])  [unwired: 2 in]
      n214 = Array Subset(array=w400, index (row)=30 ("index"), length (row)=8 ("length")) -> (w389:dbl[][])  [unwired: 2 in]
      n215 = property on="PumpSeq 4" class="Arr (strict)"("Val(Sgnl)"=w407) -> ()  [unwired: 2 in, 2 out]
      n216 = property on="PumpSeq 2" class="Arr (strict)"("Val(Sgnl)"=w402) -> ()  [unwired: 2 in, 2 out]
      n217 = property on="PumpSeq 3" class="Arr (strict)"("Val(Sgnl)"=w401) -> ()  [unwired: 2 in, 2 out]
      n218 = Index Array(array=w389, index (row)=2, index (col)=0 ("disabled index (col)")) -> ()  [unwired: 1 out]
      n219 = Index Array(array=w389, index (row)=4, index (col)=0 ("disabled index (col)")) -> ()  [unwired: 1 out]
      n220 = Index Array(array=w389, index (row)=0, index (col)=1 ("disabled index (col)")) -> ()  [unwired: 1 out]
      n221 = Index Array(array=w389, index (row)=1, index (col)=1 ("disabled index (col)")) -> ()  [unwired: 1 out]
    }
    n222 = Merge Signals(w203, w204, w72) -> (w106:dynamicdata)
    n223 = call "Build Table"("Include time data"=TRUE, "Signals"=w106) -> ("Table"=w292:string[][])  [unwired: 3 in, 6 out]
    n224 = And(x="?", y="?") -> (x .and. y?=w61:bool)
    n225 = dll-call lib="C:/Users/shresplab/OneDrive - Kemira Oyj/Documents/GitHub/Bertta/BERTTA/x64/Debug/BERTTA.dll" fn="mettler"("port"="Scale port", "msg"=1) -> ("return type"=w54:dbl)  [unwired: 5 in, 2 out]
    n226 = And(x="MASTER CONTROL", y=w61) -> (x .and. y?=w57:bool)
    n227 = Initialize Array(FALSE, 1 ("dimension size")) -> (w59:bool[])
    n228 = Replace Array Subset(array=w59, new element=w57, index=0) -> (w56:bool[])
    n229 = call "Convert to Dynamic Data5"("Double"=w54) -> ("Dynamic Data Type"=→"Waveform Chart 15":dynamicdata)  [unwired: 3 in]
    n230 = Delete From Array(array=w292, length=13, index (col)=0 ("index (row)")) -> (array with subset deleted=→"Table":string[][])  [unwired: 1 in, 1 out]
    n231 = call "DAQ Assistant"("data"=w56, "device name"="PAM Control") -> ()  [unwired: 16 in, 2 out]
    n232 = call "filenameparser_09.vi"("Description"="Description", "start path"="Browse folder", "Project name"="Project name", "User (initials)"="User (initials)", "OK Button in"="OK Button 2") -> ("appended path 2"=w147:path, "appended path"=w288:path)  [unwired: 4 in, 1 out]
    "Output File" <- w147
    n233 = Boolean To (0,1)(Boolean="OK Button") -> (0, 1=w287:i16)
    n234 = for {
      N: w287 -> [_]
      tunnel: w288 -> [w379]
      w383 = " " ("string")
      n235 = property on="Add comment" class="Str"("Val(Sgnl)"="" ("Value (Signaling)")) -> ()  [unwired: 2 in, 2 out]
      n236 = Get Date/Time String(want seconds? (F)=TRUE) -> (date string=w386:string, time string=w384:string)  [unwired: 2 in]
      n237 = Concatenate Strings(w386, w383, w384, w383, "Add comment") -> (w382:string)
      n238 = feedback #10() -> (w381:string[])  [unwired: 1 in]
      n239 = Build Array (concatenate)(w381, w382) -> (w380:string[])
      n240 = feedback-in #10(w380) -> ()
      n241 = Write to Text File(file (use dialog)=w379, text=w380) -> ()  [unwired: 2 in, 3 out]
    }
    n242 = call "Header Names 4.vi"("Dynamic Data"=w106) -> ("Signals Out"=w107:dynamicdata)  [unwired: 10 in]
    n243 = call "Write To Measurement File"("Signals"=w107, "Enable"="OK Button 2", "Filename"=w147) -> ()  [unwired: 14 in, 3 out]
    "Boolean" <- "OK Button 2"
  }
